vi "test.vi"() -> ()   [LabVIEW 2010, in "RoiGeneric.lvclass"]
uses:
  RoiGeneric.lvclass
  roi_type_enum.ctl
  common/classes/ImageCollection/ImageCollection/ImageCollection.lvclass
  common/classes/Image/Image/Image.lvclass
  RoiEllipsoid/RoiEllipsoid.lvclass
  common/classes/SpaceVector/SpaceVector/SpaceVector.lvclass
panel:
  out "x":dbl[unit]
  out "z":dbl[unit]
  out "y":dbl[unit]
  in  "ROI type":T1
  in  "depth":dbl[unit]
  in  "width":dbl[unit]
  in  "length":dbl[unit]
  out "Image":T2(plugin-control)
  in  "depth":dbl[unit](slide)
  in  "quit":bool
  in  "load image":bool
  # "Test VI for ROIGeneric"
  # "Calibration"
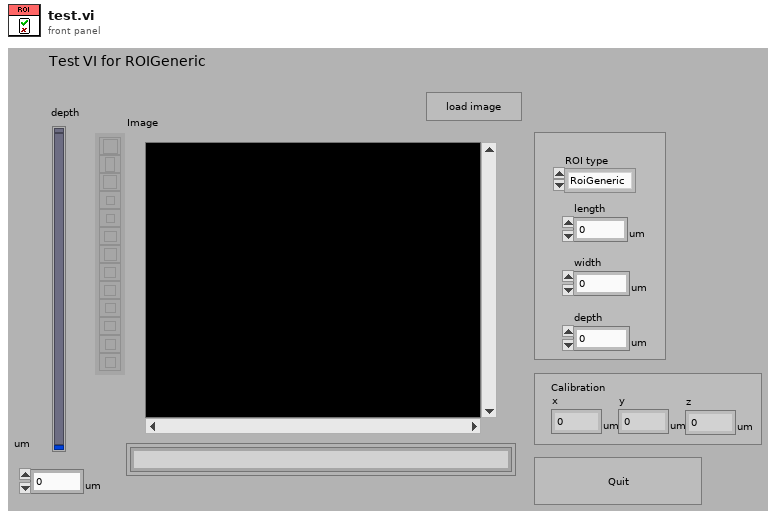
[diagram p1: front panel]
types:
  T1 = typedef "RoiGeneric.lvclass/roi_type_enum.ctl" = enum16{"RoiGeneric", "RoiEllipsoid"}
  T2 = typedef "IMAQ Image.ctl" = refnum<image>
  T3 = typedef "Image Type" = u32
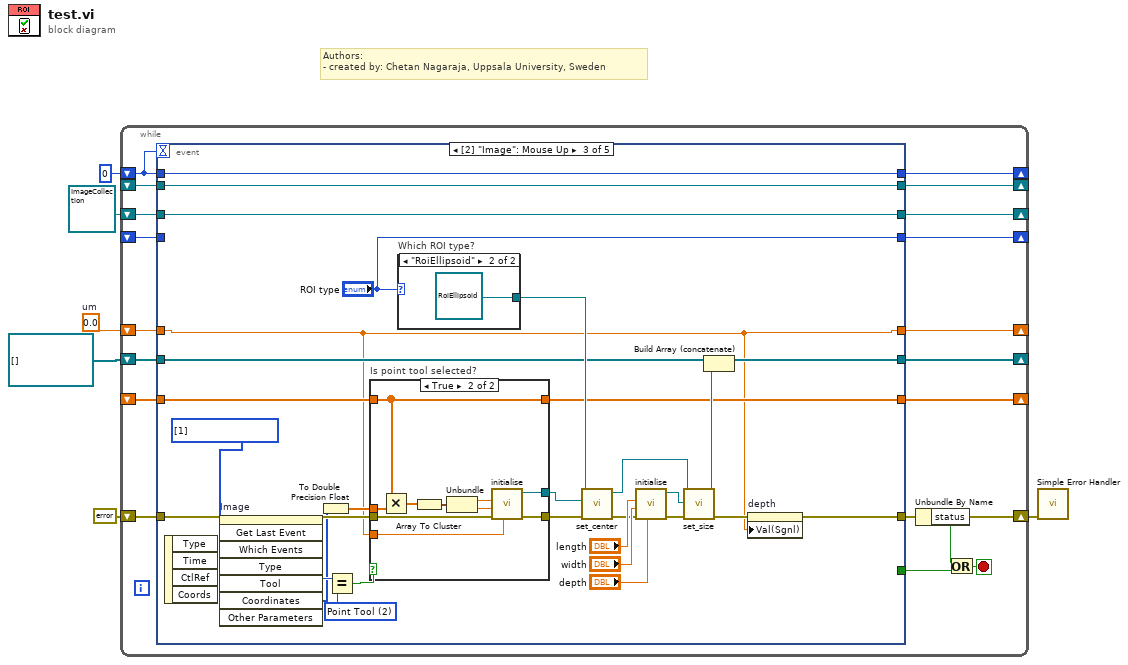
[diagram p0: block diagram]
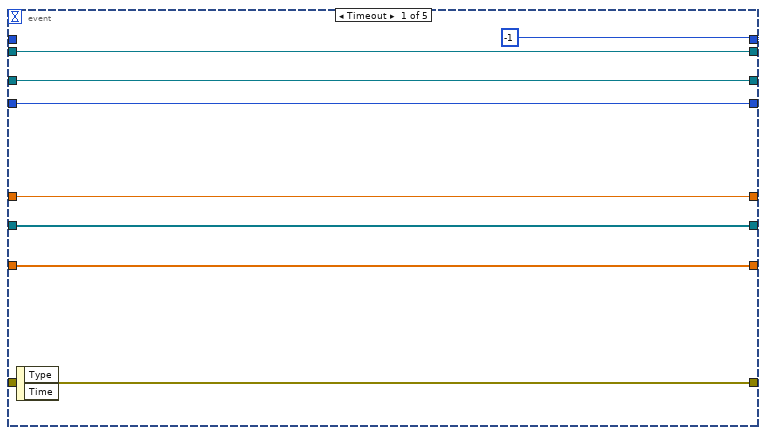
[diagram p2: hidden frame]
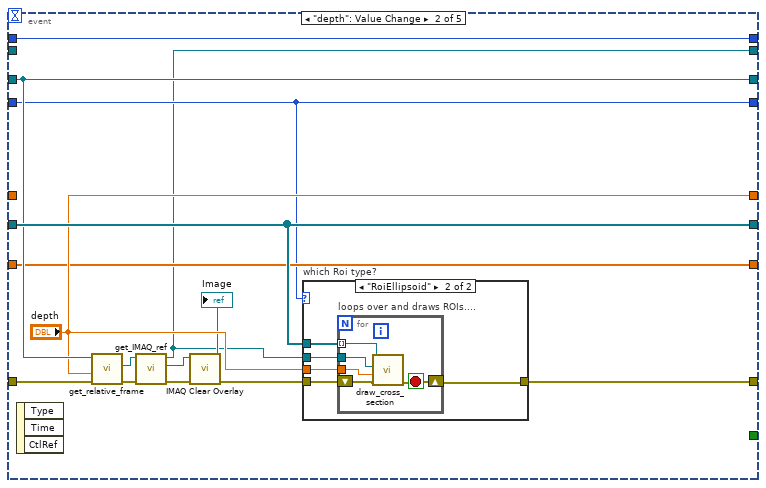
[diagram p3: hidden frame]
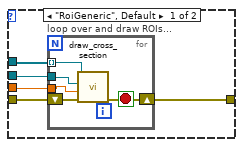
[diagram p4: hidden frame]
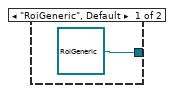
[diagram p5: hidden frame]
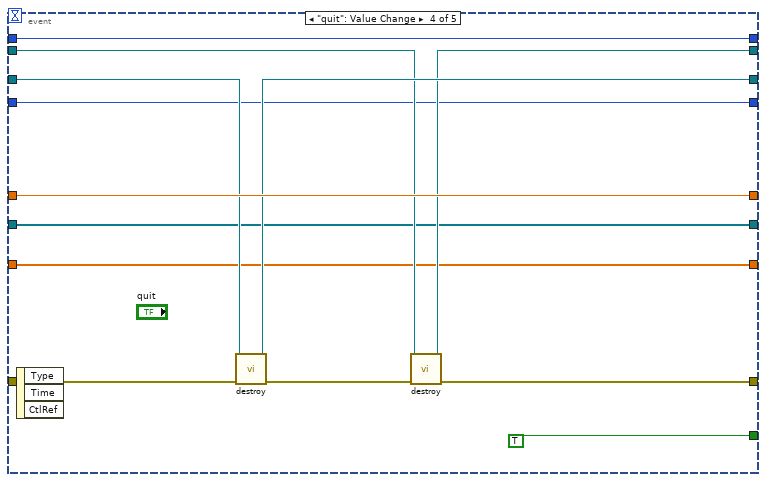
[diagram p7: hidden frame]
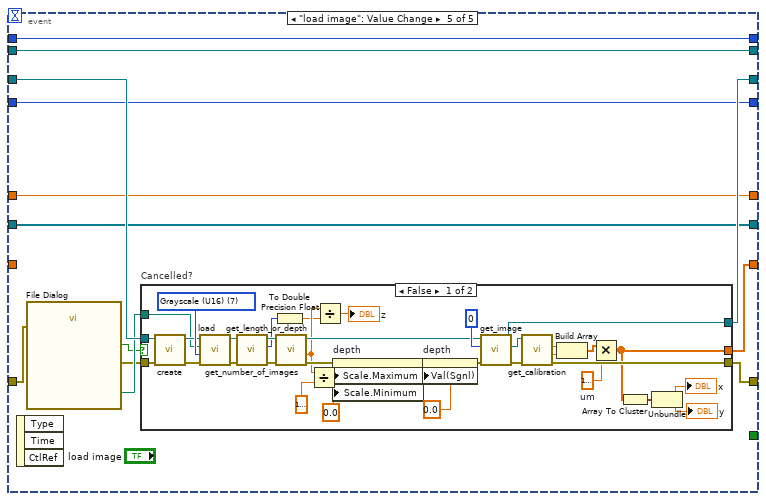
[diagram p8: hidden frame]
diagram:
  w3 = dbl[unit] 0.0  # um
  # "Authors: \n- created by: Chetan Nagaraja, Uppsala University, Sweden"
  n1 = while {
    shift-right: [w24] -> _
    shift-left: refnum<class "ImageCollection.lvclass"> refnum ("ImageCollection.lvclass") -> [w25]
    shift-right: [w22] -> _
    shift-left: w3 -> [w23]
    shift-right: [w20] -> _
    shift-left: 0 -> [w19]
    shift-right: [w18] -> _
    shift-left: _ -> [w17]
    shift-right: [w15] -> _
    shift-left: refnum<class "RoiGeneric.lvclass">[] [] -> [w16]
    shift-right: [w10] -> _
    shift-left: _ -> [w9]
    shift-right: [w14] -> w1
    shift-left: errorcluster {"status"=FALSE, "code"=0, "source"=""} ("error in") -> [w21]
    shift-right: [w8] -> _
    shift-left: _ -> [w7]
    stop <- w11 stop-if-true
    n2 = event shown="[2] \"Image\": Mouse Up" {
      selector: _ -> [_ _ _ _ _]
      dyn-events: _ -> [_ _ _ _ _]
      timeout: w19 -> [_ _ _ _ _]
      tunnel: w25 -> [w32 w42 w98 w123 w138]
      tunnel: [w32 w42 w98 w122 w136] -> w24
      tunnel: [w30 w46 w71 w119 w133] -> w14
      tunnel: w23 -> [w33 _ w69 w125 w135]
      tunnel: [w33 "depth" w69 w125 w135] -> w22
      tunnel: w21 -> [w30 w45 w93 w121 w127]
      tunnel: w19 -> [_ w48 w97 w124 w134]
      tunnel: [-1 w48 w97 w124 w134] -> w20
      tunnel: [w29 w34 w96 w117 w132] -> w18
      tunnel: w17 -> [w29 _ w96 w118 w132]
      tunnel: w16 -> [w28 w47 w77 w116 w129]
      tunnel: [w28 w47 w81 w116 w129] -> w15
      tunnel: [_ _ _ TRUE _] -> w12
      tunnel: [w27 w40 w73 w114 w128] -> w10
      tunnel: w9 -> [w27 w40 w76 w114 _]
      tunnel: [w26 w39 "ROI type" w113 w126] -> w8
      tunnel: w7 -> [w26 w39 _ w113 w126]
      event Timeout {
        n3 = event-data() -> ()  [unwired: 1 in, 2 out]
      }
      event "depth": Value Change {
        n4 = event-data() -> ()  [unwired: 1 in, 3 out]
        n5 = call-dynamic "get_relative_frame.vi"("error in (no error)"=w45, "relative depth"="depth", "ImageCollection in"=w42) -> ("error out"=w44:errorcluster, "frame"=w43:refnum<class "Image.lvclass">)  [unwired: 5 in, 2 out]
        n6 = call-dynamic "get_IMAQ_ref.vi"("error in (no error)"=w44, "Image.lvclass in"=w43) -> ("error out"=w36:errorcluster, "Image"=w38:T2, "Image.lvclass out"=w34:refnum<class "Image.lvclass">)  [unwired: 5 in, 2 out]
        n7 = call "IMAQ Clear Overlay"("error in (no error)"=w36, "Image"=w38) -> ("error out"=w35:errorcluster, "Image Out"=→"Image":T2)  [unwired: 8 in]
        n8 = case "which Roi type?" shown="\"RoiEllipsoid\"" w39 {
          tunnel: w47 -> [w53 w61]
          tunnel: w34 -> [w52 w60]
          tunnel: w35 -> [w51 w63]
          tunnel: [w50 w62] -> w46
          tunnel: "depth" -> [w49 w59]
          frame "RoiGeneric", Default {
            n9 = for "loop over and draw ROIs..." {
              shift-right: [w57] -> w50
              shift-left: w51 -> [w58]
              tunnel: w49 -> [w54]
              tunnel: w52 -> [w55]
              tunnel: w53 -> [w56] mode=indexing
              stop <- w57 stop-if-true
              n10 = call-dynamic "draw_cross_section.vi"("error in (no error)"=w58, "depth"=w54, "Image.lvclass"=w55, "RoiGeneric in"=w56) -> ("error out"=w57:errorcluster)  [unwired: 6 in, 1 out]
            }
          }
          frame "RoiEllipsoid" {
            n11 = for "loops over and draws ROIs...." {
              shift-right: [w64] -> w62
              shift-left: w63 -> [w68]
              tunnel: w61 -> [w67] mode=indexing
              tunnel: w60 -> [w66]
              tunnel: w59 -> [w65]
              stop <- w64 stop-if-true
              n12 = call-dynamic "draw_cross_section.vi"("error in (no error)"=w68, "depth"=w65, "Image.lvclass"=w66, "RoiGeneric in"=w67) -> ("error out"=w64:errorcluster)  [unwired: 6 in, 1 out]
            }
          }
        }
      }
      event "Image": Mouse Up {
        w95 = 2 items=["None", "Selection Tool", "Point Tool", "Line Tool", "Rectangle Tool", "Oval Tool", "Polygon Tool", "ClosedFreehandTool", "Annulus Tool", "Rotated Rectangle Tool", "Zoom Tool", "Pan Tool", "Polyline Tool", "Freehand Tool"] ("Tool")
        w79 = i32[] [1] items=["No Event"=0, "Click Event"=1, "Draw Event"=2, "Size Event"=4, "Scroll Event"=5, "Double Click Event"=8]
        n13 = event-data() -> ()  [unwired: 1 in, 4 out]
        n14 = invoke on="Image" class="ImageControl" method="Get Last Event"(error in=w93, "Which Events"=w79) -> (error out=w94:errorcluster, "Tool"=w92:i32, "Coordinates"=w75:i32[])  [unwired: 6 in, 5 out]
        n15 = To Double Precision Float(number=w75) -> (double precision float=w74:dbl[])
        n16 = Equal?(x=w92, y=w95) -> (x = y?=w78:bool)
        n17 = case "Is point tool selected?" shown="True" w78 {
          tunnel: w74 -> [_ w108]
          tunnel: w69 -> [_ w109]
          tunnel: w94 -> [w102 w112]
          tunnel: [w102 w111] -> w84
          tunnel: [_ w110] -> w89
          tunnel: w76 -> [w101 w103]
          tunnel: [w101 w103] -> w73
          frame False {
          }
          frame True {
            n18 = Multiply(x=w103, y=w108) -> (x*y=w107:dbl[unit][])
            n19 = Array To Cluster(array=w107) -> (cluster=w106:cluster{"[0]":dbl[unit], "[1]":dbl[unit]})
            n20 = Unbundle(w106) -> ("[0]"=w105:dbl[unit], "[1]"=w104:dbl[unit])
            n21 = call "initialise.vi"("z"=w109, "error in (no error)"=w112, "y"=w104, "x"=w105) -> ("error out"=w111:errorcluster, "SpaceVector out"=w110:refnum<class "SpaceVector.lvclass">)  [unwired: 6 in]
          }
        }
        n22 = case "Which ROI type?" shown="\"RoiEllipsoid\"" "ROI type" {
          tunnel: [refnum<class "RoiGeneric.lvclass"> refnum ("RoiGeneric.lvclass") refnum<class "RoiEllipsoid.lvclass"> refnum ("RoiEllipsoid.lvclass")] -> w91
          frame "RoiGeneric", Default {
          }
          frame "RoiEllipsoid" {
          }
        }
        n23 = call-dynamic "set_center.vi"("error in (no error)"=w84, "center"=w89, "RoiGeneric in"=w91) -> ("error out"=w83:errorcluster, "RoiGeneric out"=w90:refnum<class "RoiGeneric.lvclass">)  [unwired: 7 in]
        n24 = call "initialise.vi"("z"="depth", "error in (no error)"=w83, "y"="width", "x"="length") -> ("error out"=w82:errorcluster, "SpaceVector out"=w85:refnum<class "SpaceVector.lvclass">)  [unwired: 6 in]
        n25 = call-dynamic "set_size.vi"("error in (no error)"=w82, "size"=w85, "RoiGeneric in"=w90) -> ("error out"=w72:errorcluster, "RoiGeneric out"=w80:refnum<class "RoiGeneric.lvclass">)  [unwired: 7 in]
        n26 = Build Array (concatenate)(w77, w80) -> (w81:refnum<class "RoiGeneric.lvclass">[])
        n27 = property on="depth" class="Slide (strict)"(error in=w72, "Val(Sgnl)"=w69) -> (error out=w71:errorcluster)  [unwired: 1 in, 1 out]
      }
      event "quit": Value Change {
        n28 = event-data() -> ()  [unwired: 1 in, 3 out]
        n29 = call-dynamic "destroy.vi"("error in (no error)"=w121, "ImageCollection in"=w123) -> ("error out"=w120:errorcluster, "ImageCollection out"=w122:refnum<class "ImageCollection.lvclass">)  [unwired: 8 in]
        n30 = call-dynamic "destroy.vi"("error in (no error)"=w120, "Image in"=w118) -> ("error out"=w119:errorcluster, "Image out"=w117:refnum<class "Image.lvclass">)  [unwired: 8 in]
      }
      event "load image": Value Change {
        n31 = event-data() -> ()  [unwired: 1 in, 3 out]
        n32 = call "File Dialog"("error in"=w127) -> ("selected path"=w137:path, "cancelled"=w130:bool, "error out"=w131:errorcluster)  [unwired: 11 in, 1 out]
        n33 = case "Cancelled?" shown="False" w130 {
          tunnel: w138 -> [w171 w174]
          tunnel: w137 -> [w169 _]
          tunnel: [w158 w174] -> w136
          tunnel: w131 -> [w168 w175]
          tunnel: [w156 w175] -> w133
          tunnel: [w144 _] -> w128
          frame False {
            w153 = dbl[unit] 1e-06  # um
            w173 = T3 7 items=["Grayscale (U8)", "Grayscale (I16)", "Grayscale (SGL)", "Complex (CSG)", "RGB (U32)", "HSL (U32)", "RGB (U64)", "Grayscale (U16)"] ("Image Type")
            n34 = call "create.vi"("error in (no error)"=w168, "ImageCollection in"=w171) -> ("error out"=w172:errorcluster, "ImageCollection out"=w170:refnum<class "ImageCollection.lvclass">)  [unwired: 8 in]
            n35 = call "load.vi"("error in (no error)"=w172, "Image Type"=w173, "path in"=w169, "ImageCollection in"=w170) -> ("error out"=w152:errorcluster, "ImageCollection out"=w150:refnum<class "ImageCollection.lvclass">)  [unwired: 3 in, 3 out]
            n36 = call-dynamic "get_number_of_images.vi"("error in (no error)"=w152, "ImageCollection in"=w150) -> ("error out"=w151:errorcluster, "size"=w140:i32, "ImageCollection out"=w149:refnum<class "ImageCollection.lvclass">)  [unwired: 7 in]
            n37 = To Double Precision Float(number=w140) -> (double precision float=w139:dbl)
            n38 = call "get_length_or_depth.vi"("error in (no error)"=w151, "ImageCollection in"=w149) -> ("error out"=w167:errorcluster, "total z depth"=w141:dbl[unit], "ImageCollection out"=w159:refnum<class "ImageCollection.lvclass">)  [unwired: 5 in, 2 out]
            n39 = Divide(x=w141, y=dbl[unit] 1e-06 ("Scale.Range:Minimum")) -> (x/y=w165:dbl)
            n40 = Divide(x=w141, y=w139) -> (x/y=→"z":dbl[unit])
            n41 = property on="depth" class="Slide (strict)"(error in=w167, "Scale.Maximum"=w165, "Scale.Minimum"=0.0 ("Scale.Range:Minimum")) -> (error out=w163:errorcluster)  [unwired: 1 in, 1 out]
            n42 = property on="depth" class="Slide (strict)"(error in=w163, "Val(Sgnl)"=dbl[unit] 0.0 ("Value (Signaling)")) -> (error out=w160:errorcluster)  [unwired: 1 in, 1 out]
            n43 = call-dynamic "get_image.vi"("error in (no error)"=w160, "index"=0, "ImageCollection in"=w159) -> ("error out"=w157:errorcluster, "Image.lvclass"=w155:refnum<class "Image.lvclass">, "ImageCollection out"=w158:refnum<class "ImageCollection.lvclass">)  [unwired: 6 in]
            n44 = call "get_calibration.vi"("error in (no error)"=w157, "Image.lvclass in"=w155) -> ("error out"=w156:errorcluster, "y"=w147:dbl, "x"=w148:dbl)  [unwired: 4 in, 3 out]
            n45 = Build Array(w148, w147) -> (w154:dbl[])
            n46 = Multiply(x=w154, y=w153) -> (x*y=w144:dbl[unit][])
            n47 = Array To Cluster(array=w144) -> (cluster=w145:cluster{"[0]":dbl[unit], "[1]":dbl[unit]})
            n48 = Unbundle(w145) -> ("[0]"=→"x":dbl[unit], "[1]"=→"y":dbl[unit])
          }
          frame True {
          }
        }
      }
    }
    n49 = Unbundle By Name(w14) -> ("status"=w13:bool)
    n50 = Or(x=w13, y=w12) -> (x .or. y?=w11:bool)
  }
  n51 = call <vilib>:"Simple Error Handler.vi"("error in (no error)"=w1) -> ()  [unwired: 4 in, 5 out]
